vi "GUI.LandingPage.vi"(8 "error in":errorcluster) -> (0 "error out":errorcluster, 3 "Setting Options":T1)   [LabVIEW 2022 SP3]
panel:
  in  "Settings Square":bool caption="Settings"
  in  "Database Square":bool caption="DB"
  in  "Chart Square":bool caption="CHART"
  in  "Home Square":bool caption="HOME"
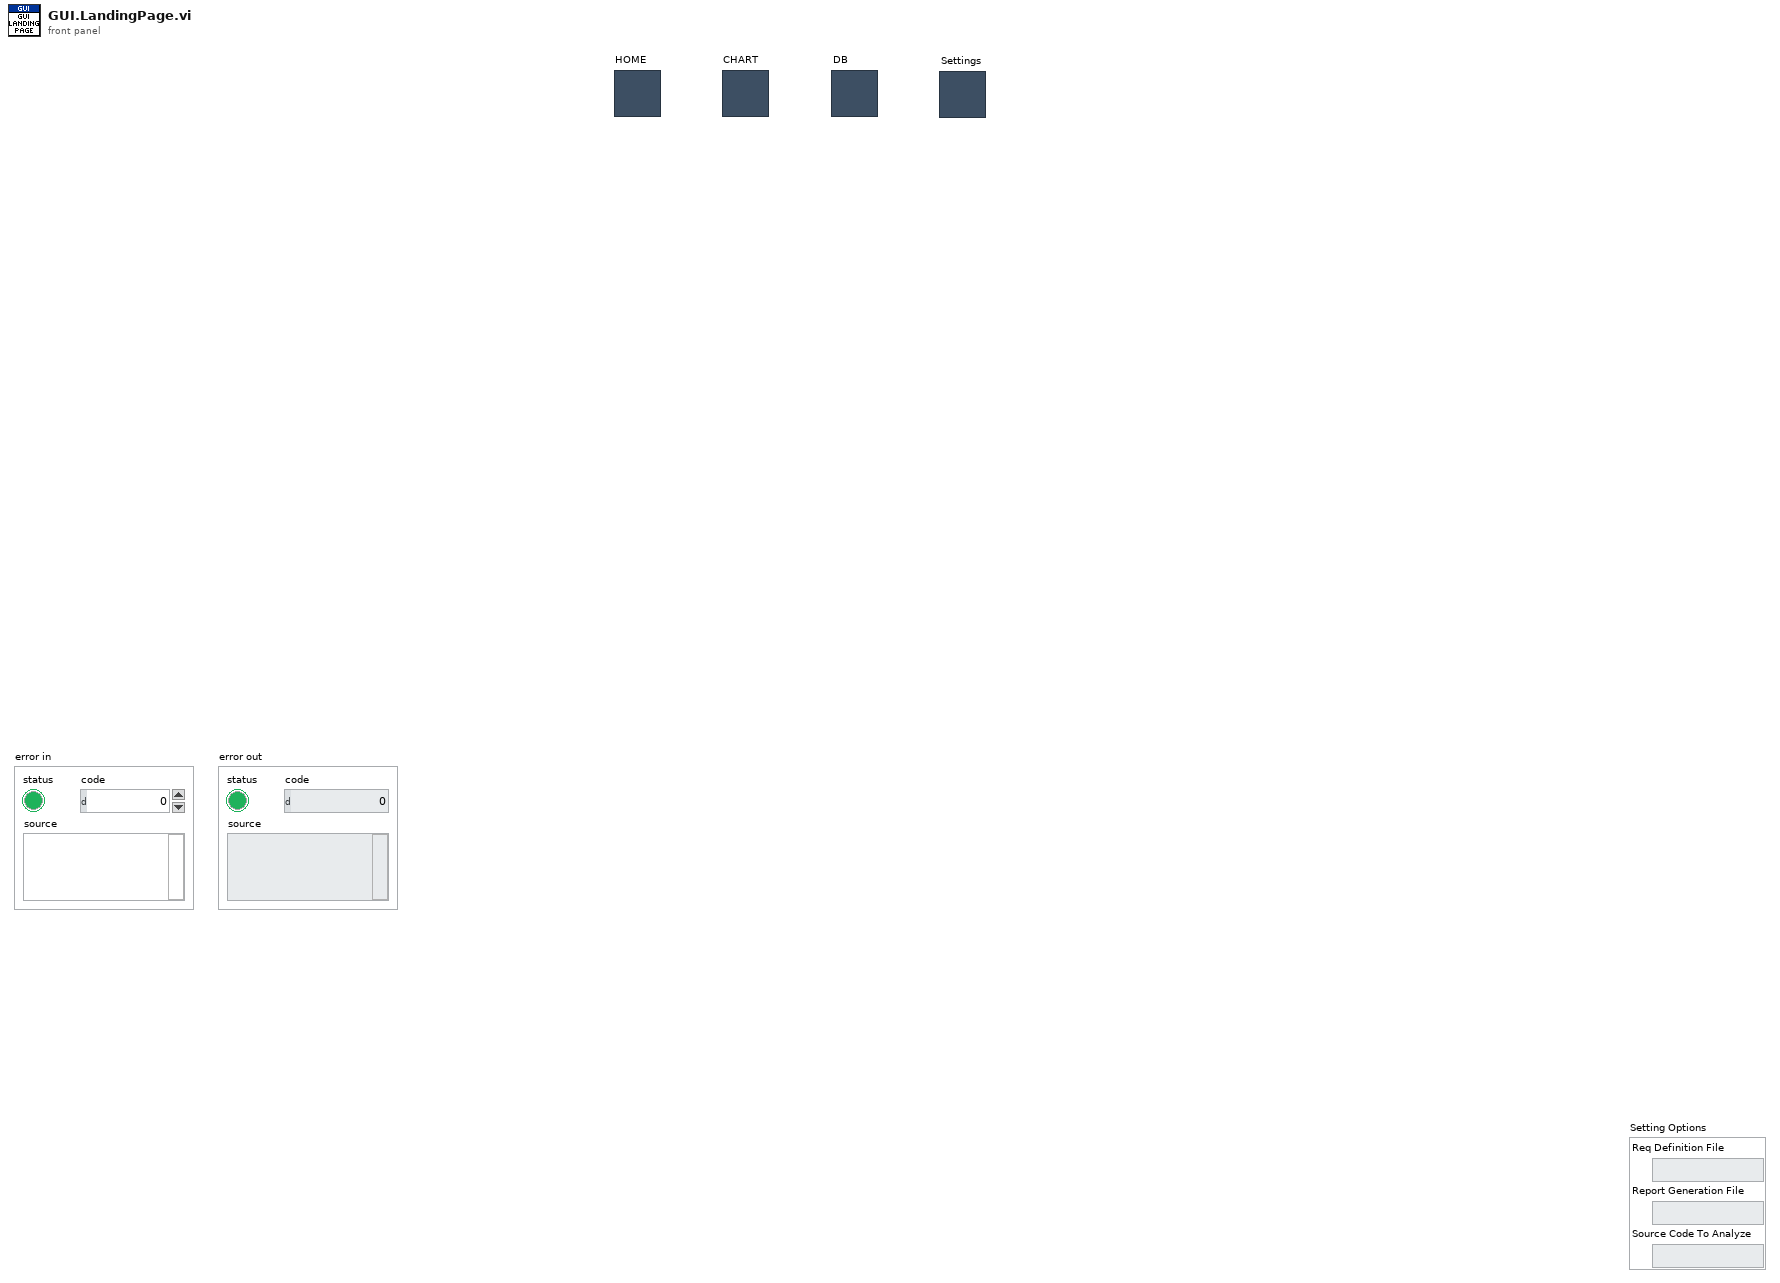
[diagram p1: front panel]
types:
  T1 = cluster{"Req Definition File":path, "Report Generation File":path, "Source Code To Analyze":path}
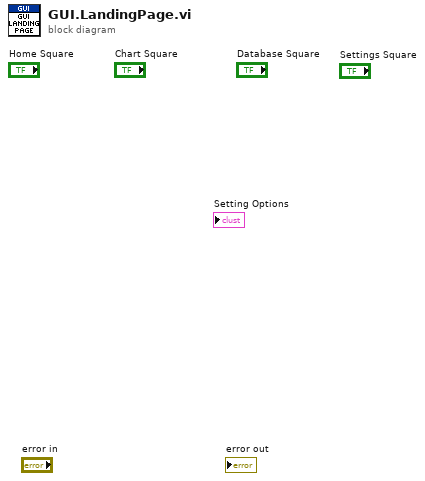
[diagram p0: block diagram]
diagram:
